vi "show_image_names.vi"() -> (3 "filenames":string[](array[string]))   [LabVIEW 2021]
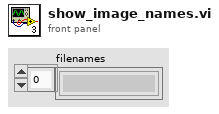
[diagram p1: front panel]
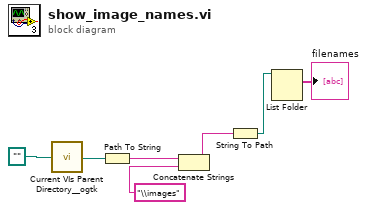
[diagram p0: block diagram]
diagram:
  n1 = call <userlib>:"Current VIs Parent Directory__ogtk.vi"("Relative path (.)"=path "") -> ("Parent Directory (+ Relative)"=w6:path)  [unwired: 4 in]
  n2 = Path To String(path=w6) -> (string=w5:string)
  n3 = Concatenate Strings(w5, "\\images") -> (w3:string)
  n4 = String To Path(string=w3) -> (path=w2:path)
  n5 = List Folder(path=w2) -> (filenames=→"filenames":string[])  [unwired: 3 in, 3 out]
